vi "Logcluster to file.vi"(0 "Log Cluster":T1, 11 "error in (no error)":errorcluster) -> (4 "CypheredText":string, 15 "error out":errorcluster)   [LabVIEW 2012]
uses:
  typedef/Log_User_Data.ctl
  typedef/User Accounts.ctl
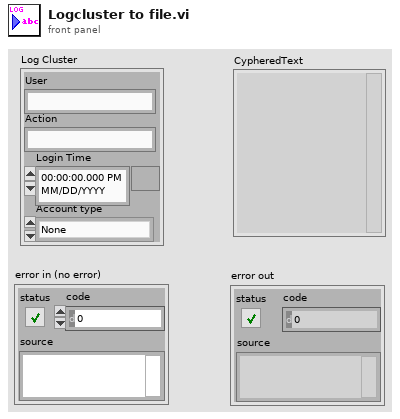
[diagram p1: front panel]
types:
  T1 = typedef "Log_User_Data.ctl" = cluster{"User":string, "Action":string, "Account type":T2, "Login Time ":timestamp}
  T2 = typedef "User Accounts.ctl" = enum16{"None", "User", "Admin"}
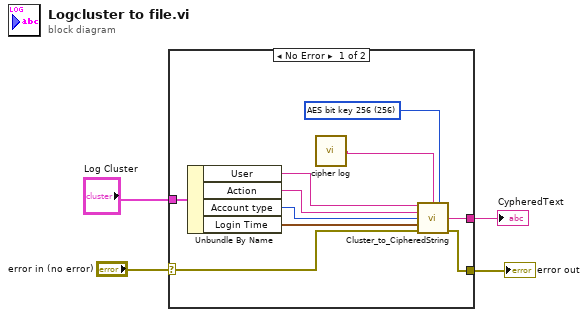
[diagram p0: block diagram]
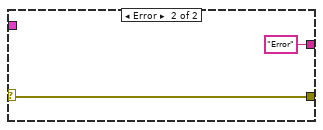
[diagram p2: hidden frame]
diagram:
  n1 = case shown="No Error" "error in (no error)" {
    selector: "error in (no error)" -> [w7 w16]
    tunnel: [w9 "Error" ("CypheredText")] -> w4
    tunnel: "Log Cluster" -> [w8 _]
    tunnel: [w6 w16] -> w1
    frame No Error {
      w10 = u16 256 items=["AES bit key 128"=128, "AES bit key 192"=192, "AES bit key 256"=256] ("BitKeyType(256)")
      n2 = Unbundle By Name(w8) -> ("User"=w14:string, "Action"=w13:string, "Account type"=w12:T2, "Login Time"=w11:timestamp)
      n3 = call "cipher log.vi"() -> ("password to cipher log"=w5:string)  [unwired: 15 in]
      n4 = call "Cluster_to_CipheredString.vi"("Usuario"=w14, "password to cipher users"=w5, "BitKeyType(256)"=w10, "Actions"=w13, "Account type"=w12, "Time Stamp"=w11, "error in (no error)"=w7) -> ("CypheredText"=w9:string, "error out"=w6:errorcluster)  [unwired: 7 in]
    }
    frame Error {
    }
  }
  "CypheredText" <- w4
  "error out" <- w1
